vi "Begin.vi"(11 "Image Size":T1=enum."160x120") -> (0 "error out":errorcluster)   [LabVIEW 2013]
doc: "Called before other user functions, this VI is expected to open initial I/O refnums, load in file data, and do all program initialization. Notice that the <B>error out</B> terminal is simply used for data flow. Wiring it to other structures or subVIs ensures that this VI runs first."
uses:
  <vilib>/Rock Robotics/WPI/Camera/WPI_CameraImageSize.ctl
  <vilib>/Rock Robotics/SystemInterfaces/DIO/FPGA_DIOPWMChannel.ctl
  <vilib>/Rock Robotics/WPI/Camera/WPI_CameraWhite Balance Values.ctl
  <vilib>/Rock Robotics/WPI/Camera/WPI_CameraExposure Values.ctl
  <vilib>/Rock Robotics/WPI/Camera/WPI_CameraFrameRate.ctl
  <vilib>/Rock Robotics/WPI/SafetyOutput/WPI_SafetyOutputConfigMenu.ctl
  <vilib>/Rock Robotics/WPI/DriverStation/WPI_DriverStationRobotMode2.ctl
  <vilib>/Rock Robotics/WPI/Joystick/WPI_JoystickDeviceEnum.ctl
  <vilib>/Rock Robotics/SystemInterfaces/DIO/FPGA_DIOChannel.ctl
  <vilib>/Rock Robotics/SystemInterfaces/DIO/FPGA_DIORelayChannel.ctl
  <vilib>/Rock Robotics/WPI/Solenoid/WPI_SolenoidChannel.ctl
  <vilib>/Rock Robotics/SystemInterfaces/Typedef/FPGA_TypedefDigitalModule.ctl
  <vilib>/Rock Robotics/SystemInterfaces/Typedef/FPGA_TypedefSolenoidModule.ctl
  <vilib>/Rock Robotics/WPI/RobotDrive/WPI_RobotDriveOpen2MotorWithJaguar.vi
  Robot Global Data.vi
  <vilib>/Rock Robotics/WPI/MotorControl/WPI_MotorControlOpen Jaguar.vi
  <vilib>/Rock Robotics/WPI/Solenoid/WPI_SolenoidOpenDouble.vi
  <vilib>/Rock Robotics/WPI/Compressor/WPI_CompressorGetSetRefNum.vi
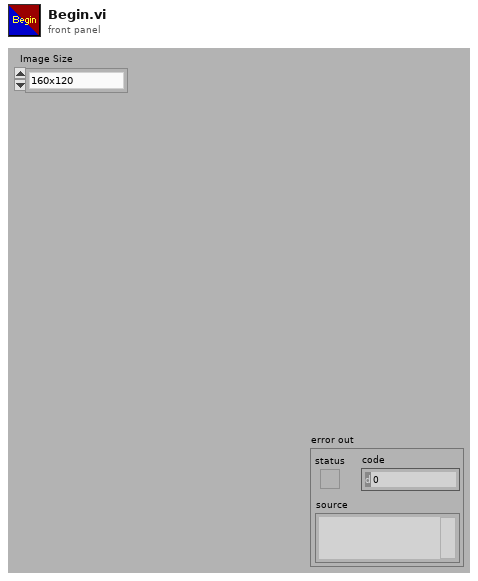
[diagram p1: front panel]
types:
  T1 = typedef "WPI_CameraImageSize.ctl" = enum16{"640x480", "320x240", "160x120"}
  T2 = typedef "WPI_JoystickDeviceEnum.ctl" = enum16{"USB 1", "USB 2", "USB 3", "USB 4", "Kinect 1", "Kinect 2"}
  T3 = typedef "FPGA_TypedefSolenoidModule.ctl" = enum16{"Solenoid Module 1", "Solenoid Module 2"}
  T4 = typedef "WPI_SolenoidChannel.ctl" = enum8{"Solenoid 1", "Solenoid 2", "Solenoid 3", "Solenoid 4", "Solenoid 5", "Solenoid 6", "Solenoid 7", "Solenoid 8", "Invalid"}
  T5 = typedef "FPGA_TypedefDigitalModule.ctl" = enum16{"Digital Module 1", "Digital Module 2"}
  T6 = typedef "FPGA_DIOPWMChannel.ctl" = enum8{"PWM 1", "PWM 2", "PWM 3", "PWM 4", "PWM 5", "PWM 6", "PWM 7", "PWM 8", "PWM 9", "PWM 10", "Invalid"}
  T7 = typedef "FPGA_DIORelayChannel.ctl" = enum8{"Relay 1", "Relay 2", "Relay 3", "Relay 4", "Relay 5", "Relay 6", "Relay 7", "Relay 8", "Invalid"}
  T8 = typedef "FPGA_DIOChannel.ctl" = enum8{"DIO 1", "DIO 2", "DIO 3", "DIO 4", "DIO 5", "DIO 6", "DIO 7", "DIO 8", "DIO 9", "DIO 10", "DIO 11", "DIO 12", "DIO 13", "DIO 14", "Invalid"}
  T9 = typedef "WPI_DriverStationRobotMode2.ctl" = enum16{"Autonomous Disabled", "Autonomous Enabled", "Teleop Disabled", "Teleop Enabled", "Timeout", "Finish", "Test Disabled", "Test Enabled"}
  T10 = typedef "WPI_SafetyOutputConfigMenu.ctl" = enum16{"Enable", "Disable"}
  T11 = typedef "WPI_CameraFrameRate.ctl" = u32
  T12 = typedef "WPI_CameraExposure Values.ctl" = enum16{"Auto", "Flicker-free 50 Hz", "Flicker-free 60 Hz", "Hold current"}
  T13 = typedef "WPI_CameraWhite Balance Values.ctl" = enum16{"Auto", "Fixed indoor", "Fixed outdoor 1", "Fixed outdoor 2", "Fixed fluorescent 1", "Fixed fluorescent 2", "Hold current"}
  T14 = typedef "WPI_SolenoidDevRef.ctl" = cluster{"DevStatus":errorcluster, "Solenoid Module":T3, "Forward Solenoid Channel":T4, "Reverse Solenoid Channel":T4}
  T15 = typedef "WPI_MotorControlDeviceRef.ctl" = cluster{"DeviceStatus":errorcluster, "Type":enum16{"PWM", "CAN"}, "PWM":cluster{"Digital Module":T5, "PWM Channel":T6, "DeadBand":T16}, "CAN":cluster{"Device Number":u8, "Control Mode":T17, "Semaphore":T18, "Max Vout":dbl}, "Invert":bool, "TransformRef":T19, "InvTransformRef":T19}
  T16 = typedef "WPI_PWMDeadband.ctl" = cluster{"Name":string, "maxPositivePwm":i32, "minPositivePwm":i32, "centerPwm":i32, "maxNegativePwm":i32, "minNegativePwm":i32, "angularRange":u16}
  T17 = typedef "WPI_CANJaguar_ControlMode.ctl" = enum8{"Percent VBus", "Current", "Speed", "Position", "Voltage"}
  T18 = typedef "Semaphore RefNum" = refnum<k1>
  T19 = typedef "WPI_PWMTransform_ConPane.ctl" = refnum<vi>
  T20 = typedef "WPI_CompressorDevRef.ctl" = cluster{"DevStatus":errorcluster, "DigitalInputDevRef":T21, "RelayDevRef":T22}
  T21 = typedef "WPI_DigitalInputDevRef.ctl" = cluster{"DevStatus":errorcluster, "DIO Channel":T8, "Digital Module":T5}
  T22 = typedef "WPI_RelayDevRef.ctl" = cluster{"DevStatus":errorcluster, "Relay Channel":T7, "Digital Module":T5, "Relay Direction":T23}
  T23 = typedef "WPI_RelayDirection.ctl" = enum16{"Both directions", "Forward only", "Reverse only"}
  T24 = typedef "WPI_CameraDevRef.ctl" = cluster{"Camera Address":string, "CameraStatus":errorcluster, "Acquire Image Notifier":refnum<notifier>}
  T25 = typedef "WPI_JoystickDevRef.ctl" = cluster{"Device":T2}
  T26 = typedef "WPI_RobotDriveDevRef.ctl" = cluster{"DevStatus":errorcluster, "Motors[]":T15[], "Square Inputs":bool, "Max Output":dbl, "Isochronous":bool}
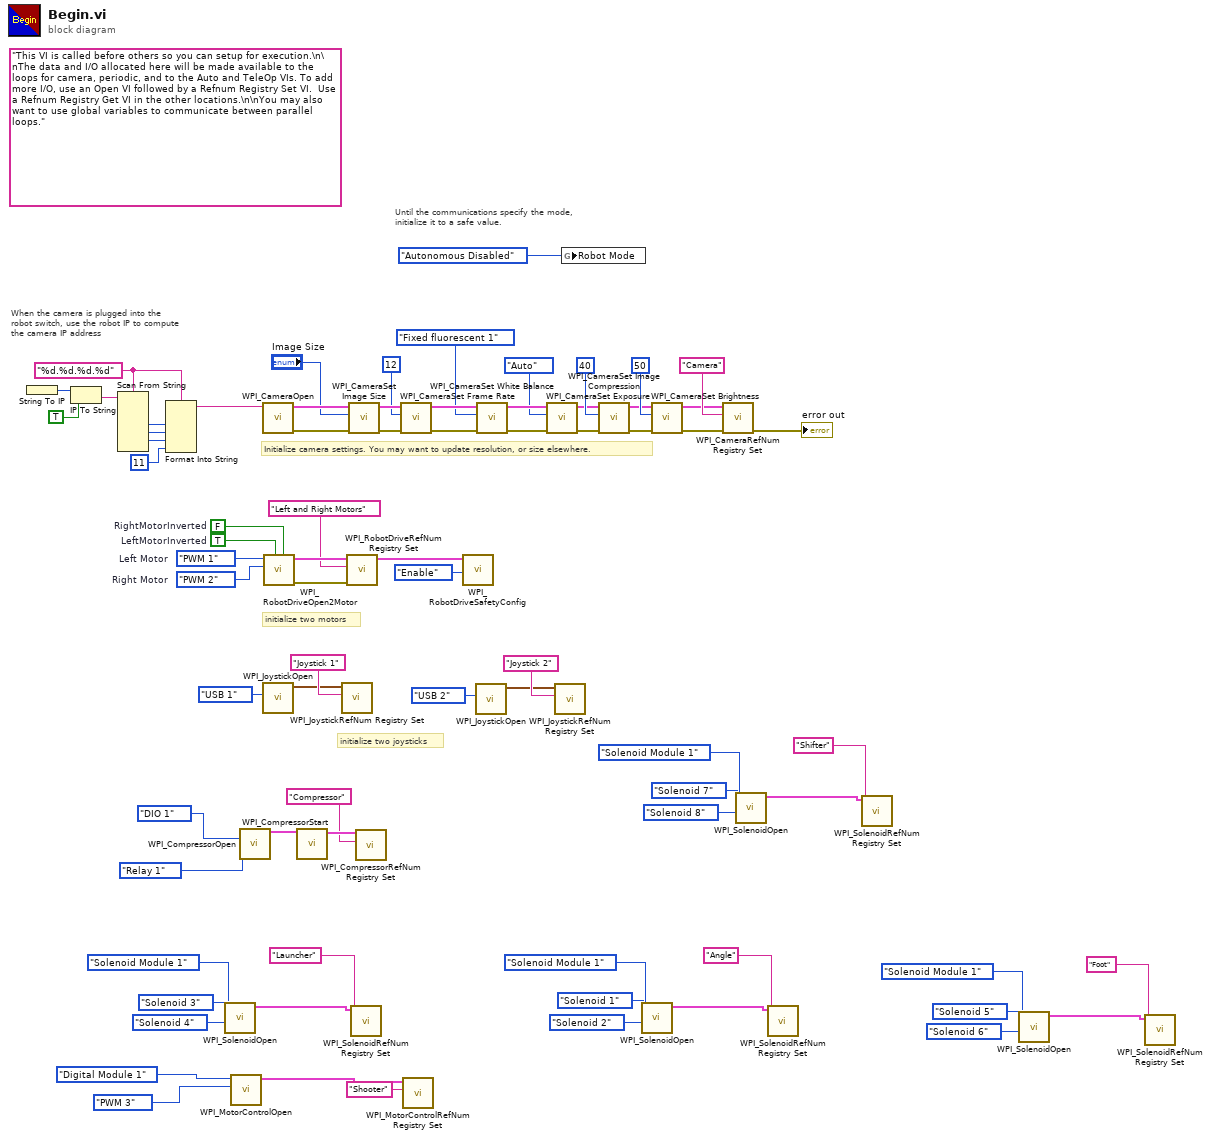
[diagram p0: block diagram]
diagram:
  w41 = "%d.%d.%d.%d" ("format string")
  (unwired) "This VI is called before others so you can setup for execution.\n\nThe data and I/O allocated here will be made available to the loops for camera, periodic, and to the Auto and TeleOp VIs. To add more I/O, use an Open VI followed by a Refnum Registry Set VI.  Use a Refnum Registry Get VI in the other locations.\n\nYou may also want to use global variables to communicate between parallel loops."
  w52 = FPGA_DIOPWMChannel."PWM 2"  # Right Motor
  w53 = FPGA_DIOPWMChannel."PWM 1"  # Left Motor
  w75 = TRUE  # LeftMotorInverted
  w76 = FALSE  # RightMotorInverted
  # "initialize two joysticks"
  # "Until the communications specify the mode,\ninitialize it to a safe value."
  # "When the camera is plugged into the\nrobot switch, use the robot IP to compute\nthe camera IP address"
  # "initialize two motors"
  # "Initialize camera settings. You may want to update resolution, or size elsewhere."
  n1 = String To IP() -> (0:w48:u32)  [unwired: 1 in]
  n2 = IP To String(1:TRUE ("dot notation? (F)"), 2:w48) -> (0:w46:string)
  n3 = Scan From String(format string=w41, input string=w46) -> (output 1=w45:i32, output 2=w44:i32, output 3=w43:i32)  [unwired: 7 in, 3 out]
  n4 = Format Into String(format string=w41, w45, w44, w43, 11 ("Compression")) -> (resulting string=w37:string)  [unwired: 2 in, 1 out]
  n5 = call-poly <vilib>:"WPI_SolenoidOpen.vi"("Reverse Solenoid Channel"=WPI_SolenoidChannel."Solenoid 4", "Forward Solenoid Channel"=WPI_SolenoidChannel."Solenoid 3", "Solenoid Module (Module 1)"=FPGA_TypedefSolenoidModule."Solenoid Module 1") -> ("SolenoidDevRef"=w24:T14)  [unwired: 7 in, 1 out]
  n6 = call-poly <vilib>:"WPI_MotorControlOpen.vi"("PWM Channel"=FPGA_DIOPWMChannel."PWM 3", "Digital Module (Module 1)"=FPGA_TypedefDigitalModule."Digital Module 1") -> ("MotorControlDeviceRef"=w23:T15)  [unwired: 8 in, 1 out]
  n7 = call <vilib>:"WPI_CompressorOpen.vi"("Pressure Switch DIO Channel"=FPGA_DIOChannel."DIO 1", "Relay Channel"=FPGA_DIORelayChannel."Relay 1") -> ("CompressorDevRef"=w32:T20)  [unwired: 12 in, 1 out]
  n8 = call <vilib>:"WPI_CameraOpen.vi"("Camera Address"=w37) -> ("error out"=w62:errorcluster, "CameraDevRef"=w63:T24)  [unwired: 1 in, 8 out]
  n9 = call <vilib>:"WPI_JoystickOpen.vi"("JoystickDevice"=WPI_JoystickDeviceEnum."USB 1") -> ("JoystickDevRef"=w35:T25)  [unwired: 10 in]
  n10 = call-poly <vilib>:"WPI_RobotDriveOpen2Motor.vi"("Right Motor Inverted"=w76, "Left Motor Inverted"=w75, "Right Motor"=w52, "Left Motor"=w53) -> ("error out"=w71:errorcluster, "RobotDriveDevRef"=w73:T26)  [unwired: 1 in, 5 out]
  n11 = call <vilib>:"WPI_CompressorStart.vi"("CompressorDevRef"=w32) -> ("CompressorDevRef"=w31:T20)  [unwired: 9 in, 1 out]
  n12 = call <vilib>:"WPI_JoystickRefNum Registry Set.vi"("refnum name"="Joystick 1", "JoystickDevRef"=w35) -> ()  [unwired: 8 in, 2 out]
  n13 = call <vilib>:"WPI_RobotDriveRefNum Registry Set.vi"("error in (no error)"=w71, "refnum name"="Left and Right Motors", "RobotDriveDevRef"=w73) -> ("RobotDriveDevRef"=w40:T26)  [unwired: 8 out]
  n14 = call <vilib>:"WPI_CameraSet Image Size.vi"("error in (no error)"=w62, "Image Size"="Image Size", "CameraDevRef"=w63) -> ("error out"=w61:errorcluster, "CameraDevRef Out"=w64:T24)  [unwired: 7 out]
  n15 = call <vilib>:"WPI_SolenoidRefNum Registry Set.vi"("refnum name"="Launcher", "SolenoidDevRef"=w24) -> ()  [unwired: 8 in, 2 out]
  n16 = call <vilib>:"WPI_CompressorRefNum Registry Set.vi"("refnum name"="Compressor", "CompressorDevRef"=w31) -> ()  [unwired: 8 in, 2 out]
  n17 = call <vilib>:"WPI_CameraSet Frame Rate.vi"("error in (no error)"=w61, "Frame Rate (fps)"=T11 12, "CameraDevRef"=w64) -> ("error out"=w60:errorcluster, "CameraDevRef Out"=w66:T24)  [unwired: 7 out]
  n18 = call <vilib>:"WPI_MotorControlRefNum Registry Set.vi"("refnum name"="Shooter", "MotorControlDevRef"=w23) -> ()  [unwired: 8 in, 2 out]
  n19 = call <vilib>:"WPI_RobotDriveSafetyConfig.vi"("mode"=WPI_SafetyOutputConfigMenu."Enable", "RobotDriveDevRef"=w40) -> ()  [unwired: 8 in, 2 out]
  n20 = call <vilib>:"WPI_JoystickOpen.vi"("JoystickDevice"=WPI_JoystickDeviceEnum."USB 2") -> ("JoystickDevRef"=w2:T25)  [unwired: 10 in]
  n21 = call <vilib>:"WPI_CameraSet White Balance.vi"("error in (no error)"=w60, "White Balance"=WPI_CameraWhite_Balance_Values."Fixed fluorescent 1", "CameraDevRef"=w66) -> ("error out"=w59:errorcluster, "CameraDevRef Out"=w65:T24)  [unwired: 7 out]
  n22 = call <vilib>:"WPI_CameraSet Exposure.vi"("error in (no error)"=w59, "Exposure"=WPI_CameraExposure_Values."Auto", "CameraDevRef"=w65) -> ("error out"=w58:errorcluster, "CameraDevRef Out"=w68:T24)  [unwired: 7 out]
  n23 = call <vilib>:"WPI_JoystickRefNum Registry Set.vi"("refnum name"="Joystick 2", "JoystickDevRef"=w2) -> ()  [unwired: 8 in, 2 out]
  n24 = global write "Robot Global Data.vi" "Robot Mode"(WPI_DriverStationRobotMode2."Autonomous Disabled" ("Robot Mode")) -> ()
  n25 = call <vilib>:"WPI_CameraSet Image Compression.vi"("error in (no error)"=w58, "Compression"=40, "CameraDevRef"=w68) -> ("error out"=w57:errorcluster, "CameraDevRef Out"=w67:T24)  [unwired: 7 out]
  n26 = call-poly <vilib>:"WPI_SolenoidOpen.vi"("Reverse Solenoid Channel"=WPI_SolenoidChannel."Solenoid 2", "Forward Solenoid Channel"=WPI_SolenoidChannel."Solenoid 1", "Solenoid Module (Module 1)"=FPGA_TypedefSolenoidModule."Solenoid Module 1") -> ("SolenoidDevRef"=w17:T14)  [unwired: 7 in, 1 out]
  n27 = call <vilib>:"WPI_CameraSet Brightness.vi"("error in (no error)"=w57, "Brightness"=50, "CameraDevRef"=w67) -> ("error out"=w55:errorcluster, "CameraDevRef Out"=w56:T24)  [unwired: 7 out]
  n28 = call <vilib>:"WPI_CameraRefNum Registry Set.vi"("error in (no error)"=w55, "refnum name"="Camera", "CameraDevRef"=w56) -> ("error out"=→"error out":errorcluster)  [unwired: 8 out]
  n29 = call-poly <vilib>:"WPI_SolenoidOpen.vi"("Reverse Solenoid Channel"=WPI_SolenoidChannel."Solenoid 8", "Forward Solenoid Channel"=WPI_SolenoidChannel."Solenoid 7", "Solenoid Module (Module 1)"=FPGA_TypedefSolenoidModule."Solenoid Module 1") -> ("SolenoidDevRef"=w7:T14)  [unwired: 7 in, 1 out]
  n30 = call <vilib>:"WPI_SolenoidRefNum Registry Set.vi"("refnum name"="Angle", "SolenoidDevRef"=w17) -> ()  [unwired: 8 in, 2 out]
  n31 = call <vilib>:"WPI_SolenoidRefNum Registry Set.vi"("refnum name"="Shifter", "SolenoidDevRef"=w7) -> ()  [unwired: 8 in, 2 out]
  n32 = call-poly <vilib>:"WPI_SolenoidOpen.vi"("Reverse Solenoid Channel"=WPI_SolenoidChannel."Solenoid 6", "Forward Solenoid Channel"=WPI_SolenoidChannel."Solenoid 5", "Solenoid Module (Module 1)"=FPGA_TypedefSolenoidModule."Solenoid Module 1") -> ("SolenoidDevRef"=w10:T14)  [unwired: 7 in, 1 out]
  n33 = call <vilib>:"WPI_SolenoidRefNum Registry Set.vi"("refnum name"="Foot", "SolenoidDevRef"=w10) -> ()  [unwired: 8 in, 2 out]
